vi "ToF Calibration (Lab).vi"() -> ()   [LabVIEW 2014]
uses:
  Type Defs/VL6180X DEFS.ctl
  <vilib>/Analysis/baseanly.llb/Mean (DBL).vi
  <vilib>/MakerHub/LINX/Public/Utilities/Open Local.vi
  <vilib>/MakerHub/LINX/LMH-LINX.lvlib
  <vilib>/Analysis/NI_AALBase.lvlib
panel:
  in  "Submit Calibration Change":bool
  in  "Offset":u8=20 format="%02x"
  out "Offset Read":u8 format="%02x"
  out "range":dbl
  out "Array":dbl[](array[numeric])
  out "min value":dbl
  out "max value":dbl
  out "mean":dbl format="%0.2f"
  in  "Samples to Avg":i32=10
  in  "Time between samples (ms)":u32=20
  out "Sensor Error Code":u8
  in  "Stop":bool
  out "Distance":u8(graph)
  # "0 = No error\n6 = early convergence estimate check failed\n7 = max convergence issue"
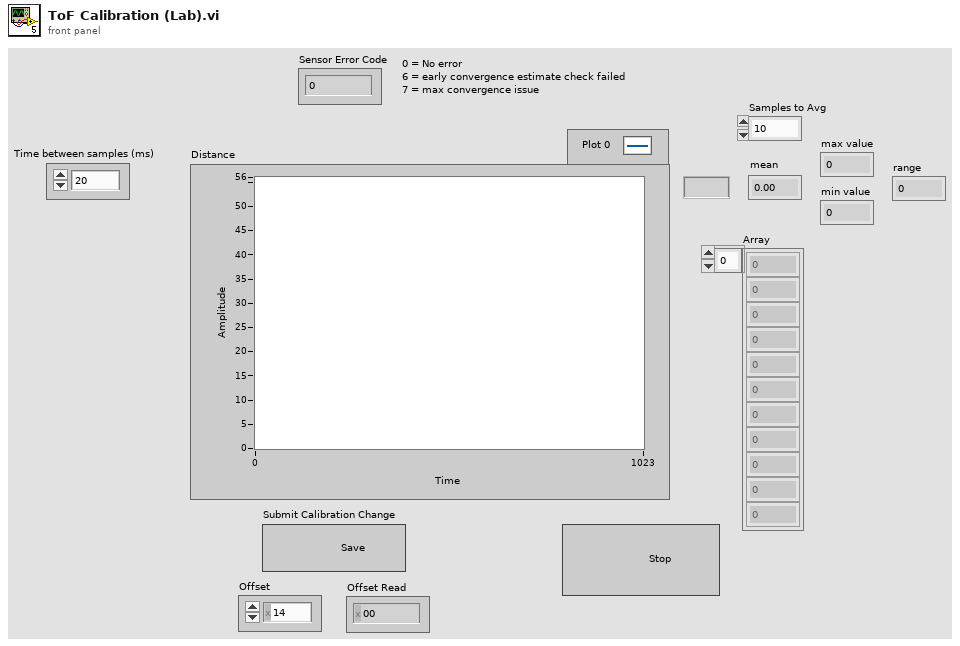
[diagram p1: front panel]
types:
  T1 = typedef "LMH-LINX.lvlib/LINX Ref.ctl" = cluster{"IO":T2, "Interface":T3, "LINX Device Config":T4}
  T2 = typedef "LMH-LINX.lvlib/Platform.ctl" = enum16{"Remote", "Local"}
  T3 = typedef "LMH-LINX.lvlib/Interface.ctl" = enum16{"Serial", "TCP"}
  T4 = typedef "LMH-LINX.lvlib/Device.lvlib/LINX Device Config.ctl" = cluster{"Interface":T3, "COM Port":refnum<visa-resource-name>, "TCP Configuration":T5, "Device Family":u8, "Device ID":u8, "Device Name":string, "TCP Ref":refnum<k5>, "Channels":T6}
  T5 = typedef "LMH-LINX.lvlib/Device.lvlib/TCP Config.ctl" = cluster{"IP Address":string, "Port":u16}
  T6 = typedef "LMH-LINX.lvlib/Channels.ctl" = cluster{"DI":u8[], "DO":u8[], "AI":u8[], "AO":u8[], "PWM":u8[], "QE":u8[], "UART":u8[], "I2C 2":u8[], "SPI":u8[], "CAN":u8[], "Servo":u8[], "AI Ref (V)":dbl, "AI Resolution (Bits)":u8, "AO Ref (V)":dbl, "AO Resolution (Bits)":u8}
  T7 = typedef "VL6180 Resource.ctl" = cluster{"LINX Resource":T1, "I2C Channel":u8, "I2C Slave Address":u8}
  T8 = typedef "VL6180X DEFS.ctl" = u16
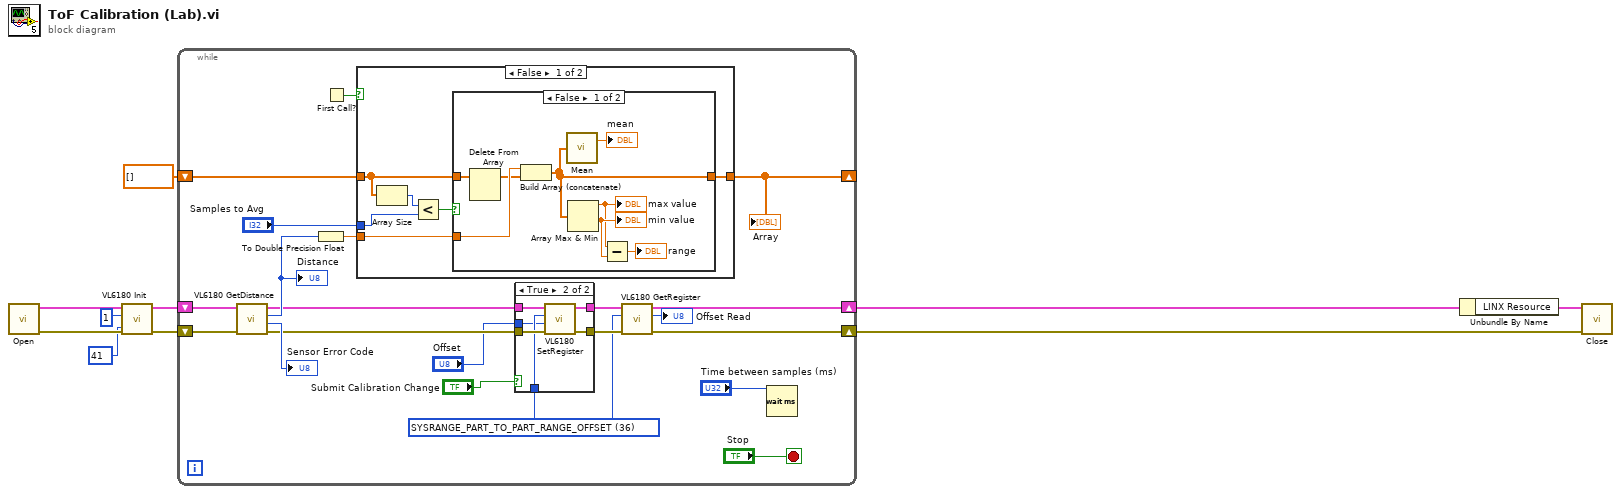
[diagram p0: block diagram]
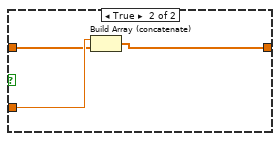
[diagram p3: hidden frame]
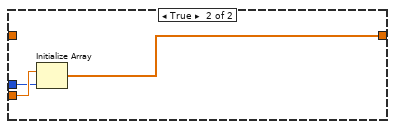
[diagram p4: hidden frame]
diagram:
  n1 = call-poly <vilib>:"Open.vi"() -> ("Error Out"=w9:errorcluster, "LINX Resource"=w10:T1)  [unwired: 9 in, 1 out]
  n2 = call "VL6180 Init.vi"("Error In"=w9, "I2C Slave Address (0)"=u8 41, "I2C Channel"=u8 1, "LINX Resource"=w10) -> ("Error Out"=w5:errorcluster, "VL6180 Resource"=w6:T7)  [unwired: 6 in]
  n3 = while {
    shift-right: [w20] -> w3
    shift-left: w6 -> [w31]
    shift-right: [w19] -> w4
    shift-left: w5 -> [w30]
    shift-right: [w22] -> _
    shift-left: dbl[] [] -> [w21]
    stop <- "Stop" stop-if-true
    w13 = T8 36 items=["IDENTIFICATION_MODEL_ID"=0, "IDENTIFICATION_MODEL_REV_MAJOR"=1, "IDENTIFICATION_MODEL_REV_MINOR"=2, "IDENTIFICATION_MODULE_REV_MAJOR"=3, "IDENTIFICATION_MODULE_REV_MINOR"=4, "IDENTIFICATION_DATE"=6, "IDENTIFICATION_TIME"=8, "SYSTEM_MODE_GPIO0"=16, "SYSTEM_MODE_GPIO1"=17, "SYSTEM_HISTORY_CTRL"=18, "SYSTEM_INTERRUPT_CONFIG_GPIO"=20, "SYSTEM_INTERRUPT_CLEAR"=21, "SYSTEM_FRESH_OUT_OF_RESET"=22, "SYSTEM_GROUPED_PARAMETER_HOLD"=23, "SYSRANGE_START"=24, "SYSRANGE_THRESH_HIGH"=25, "SYSRANGE_THRESH_LOW"=26, "SYSRANGE_INTERMEASUREMENT_PERIOD"=27, "SYSRANGE_MAX_CONVERGENCE_TIME"=28, "SYSRANGE_CROSSTALK_COMPENSATION_RATE"=30, "SYSRANGE_CROSSTALK_VALID_HEIGHT"=33, "SYSRANGE_EARLY_CONVERGENCE_ESTIMATE"=34, "SYSRANGE_PART_TO_PART_RANGE_OFFSET"=36, "SYSRANGE_RANGE_IGNORE_VALID_HEIGHT"=37, "SYSRANGE_RANGE_IGNORE_THRESHOLD"=38, "SYSRANGE_MAX_AMBIENT_LEVEL_MULT"=44, "SYSRANGE_RANGE_CHECK_ENABLES"=45, "SYSRANGE_VHV_RECALIBRATE"=46, "SYSRANGE_VHV_REPEAT_RATE"=49, "SYSALS_START"=56, "SYSALS_THRESH_HIGH"=58, "SYSALS_THRESH_LOW"=60, "SYSALS_INTERMEASUREMENT_PERIOD"=62, "SYSALS_ANALOGUE_GAIN"=63, "SYSALS_INTEGRATION_PERIOD"=64, "RESULT_RANGE_STATUS"=77, "RESULT_ALS_STATUS"=78, "RESULT_INTERRUPT_STATUS_GPIO"=79, "RESULT_ALS_VAL"=80, "RESULT_HISTORY_BUFFER"=82, "RESULT_RANGE_VAL"=98, "RESULT_RANGE_RAW"=100, "RESULT_RANGE_RETURN_RATE"=102, "RESULT_RANGE_REFERENCE_RATE"=104, "RESULT_RANGE_RETURN_SIGNAL_COUNT"=108, "RESULT_RANGE_REFERENCE_SIGNAL_COUNT"=112, "RESULT_RANGE_RETURN_AMB_COUNT"=116, "RESULT_RANGE_REFERENCE_AMB_COUNT"=120, "RESULT_RANGE_RETURN_CONV_TIME"=124, "RESULT_RANGE_REFERENCE_CONV_TIME"=128, "READOUT_AVERAGING_SAMPLE_PERIOD"=266, "FIRMWARE_BOOTUP"=281, "FIRMWARE_RESULT_SCALER"=288, "I2C_SLAVE_DEVICE_ADDRESS"=530, "INTERLEAVED_MODE_ENABLE"=675] ("VL6180X Constants")
    n4 = call "VL6180 GetDistance.vi"("error in (no error)"=w30, "VL6180 Resource in"=w31) -> ("error out"=w16:errorcluster, "Sensor Error Code"=→"Sensor Error Code":u8, "Distance (mm)"=w25:u8, "VL6180 Resource out"=w17:T7)  [unwired: 6 in]
    "Distance" <- w25
    n5 = To Double Precision Float(number=w25) -> (double precision float=w24:dbl)
    n6 = First Call?() -> (First Call?: T/F=w26:bool)
    n7 = case shown="False" w26 {
      tunnel: w24 -> [w42 w59]
      tunnel: "Samples to Avg" -> [w43 w58]
      tunnel: [w40 w57] -> w22
      tunnel: w21 -> [w41 _]
      frame False {
        n8 = Array Size(array=w41) -> (size(s)=w44:i32)
        n9 = Less?(x=w44, y=w43) -> (x < y?=w45:bool)
        n10 = case shown="False" w45 {
          tunnel: w42 -> [w52 w56]
          tunnel: w41 -> [w53 w55]
          tunnel: [w50 w54] -> w40
          frame False {
            n11 = Delete From Array(array=w53) -> (array with subset deleted=w51:dbl[])  [unwired: 2 in, 1 out]
            n12 = Build Array (concatenate)(w52, w51) -> (w50:dbl[])
            n13 = call-poly <vilib>:"Mean.vi"("X"=w50) -> ("mean"=→"mean":dbl)  [unwired: 1 out]
            n14 = Array Max & Min(array=w50) -> (max value=w47:dbl, min value=w48:dbl)  [unwired: 2 out]
            "max value" <- w47
            "min value" <- w48
            n15 = Subtract(x=w47, y=w48) -> (x-y=→"range":dbl)
          }
          frame True {
            n16 = Build Array (concatenate)(w56, w55) -> (w54:dbl[])
          }
        }
      }
      frame True {
        n17 = Initialize Array(w59, w58) -> (w57:dbl[])
      }
    }
    "Array" <- w22
    n18 = case shown="True" "Submit Calibration Change" {
      tunnel: w17 -> [w33 w39]
      tunnel: w16 -> [w32 w38]
      tunnel: [w33 w37] -> w15
      tunnel: [w32 w36] -> w14
      tunnel: w13 -> [_ w35]
      tunnel: "Offset" -> [_ w34]
      frame False {
      }
      frame True {
        n19 = call "VL6180 SetRegister.vi"("error in (no error)"=w38, "Data in"=w34, "Address"=w35, "VL6180 Resource"=w39) -> ("error out"=w36:errorcluster, "VL6180 Resource"=w37:T7)  [unwired: 6 in]
      }
    }
    n20 = call "VL6180 GetRegister.vi"("error in"=w14, "VL6180X Constants"=w13, "VL6180 Resource"=w15) -> ("error out"=w19:errorcluster, "Data out"=→"Offset Read":u8, "VL6180 Resource"=w20:T7)  [unwired: 6 in]
    n21 = Wait (ms)(milliseconds to wait="Time between samples (ms)") -> ()  [unwired: 1 out]
  }
  n22 = Unbundle By Name(w3) -> ("LINX Resource"=w2:T1)
  n23 = call <vilib>:"Close.vi"("Error In"=w4, "LINX Resource"=w2) -> ()  [unwired: 9 in, 1 out]
